vi "y1y2 (子VI)备份.vi"(0 "Image Pixels (U8)输入":u8[][](array[numeric])) -> (7 "left":cluster{i32, i32}[](graph), 8 "right":cluster{i32, i32}[](graph))   [LabVIEW 2014]
panel:
  out "Image Pixels (U8)输入 2":u8[][](array[numeric])
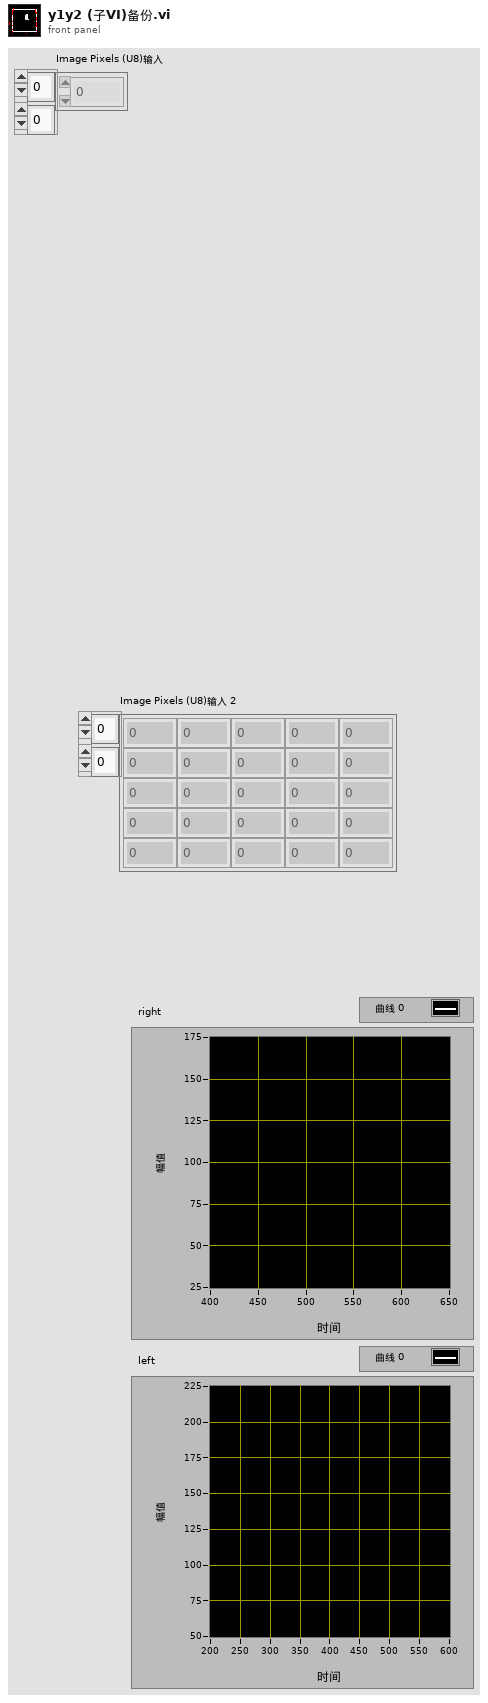
[diagram p1: front panel]
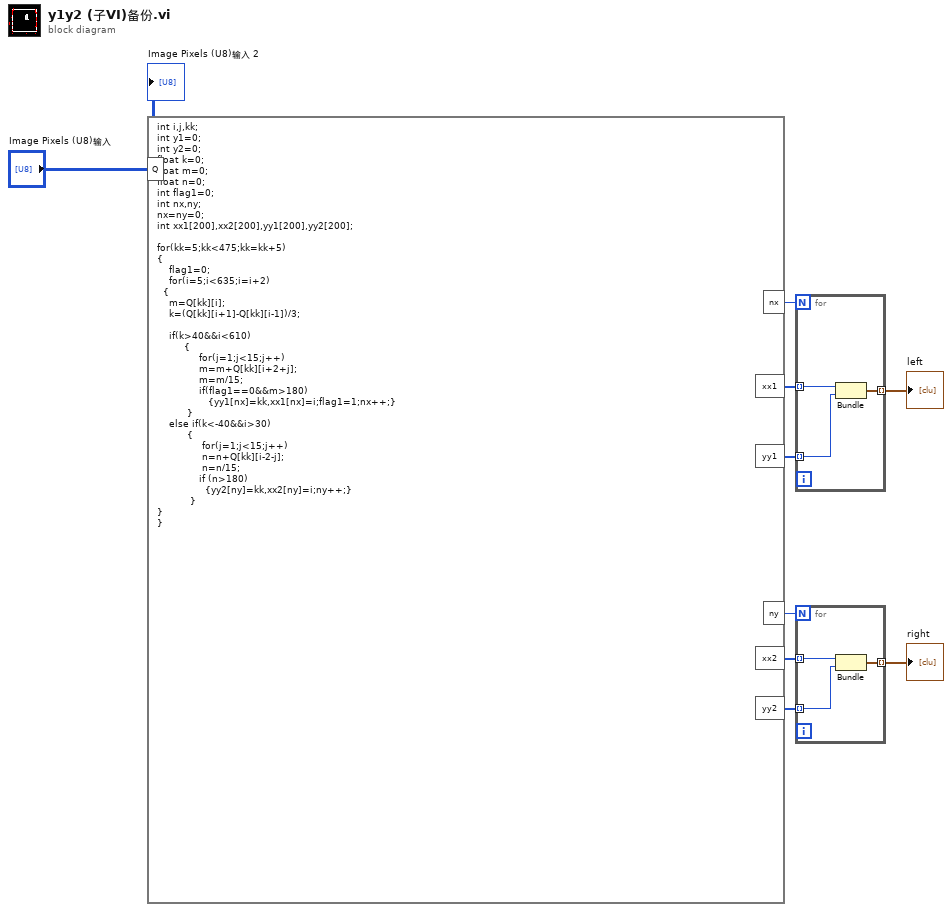
[diagram p0: block diagram]
diagram:
  n1 = formula code="int i,j,kk;\nint y1=0;\nint y2=0;\nfloat k=0;\nfloat m=0;\nfloat n=0;\nint flag1=0;\nint nx,ny;\nnx=ny=0;\nint xx1[200],xx2[200],yy1[200],yy2[200];\n\nfor(kk=5;kk<475;kk=kk+5)\n{\n    flag1=0;\n    for(i=5;i<635;i=i+2)\n  {\n    m=Q[kk][i];\n    k=(Q[kk][i+1]-Q[kk][i-1])/3;\n\n    if(k>40&&i<610)\n         {   \n              for(j=1;j<15;j++)\n              m=m+Q[kk][i+2+j];\n              m=m/15;\n              if(flag1==0&&m>180)\n                 {yy1[nx]=kk,xx1[nx]=i;flag1=1;nx++;}\n          }\n    else if(k<-40&&i>30)\n          {                   \n               for(j=1;j<15;j++)\n               n=n+Q[kk][i-2-j];\n               n=n/15;\n              if (n>180)\n                {yy2[ny]=kk,xx2[ny]=i;ny++;}\n           }\n}\n}"("Q"="Image Pixels (U8)输入") -> ("xx1"=w2:i32[], "yy1"=w1:i32[], "nx"=w3:i32, "xx2"=w4:i32[], "yy2"=w5:i32[], "ny"=w8:i32)
  n2 = for {
    N: w3 -> [_]
    tunnel: w2 -> [w12] mode=indexing
    tunnel: w1 -> [w11] mode=indexing
    tunnel: [w10] -> w6 mode=indexing
    n3 = Bundle(w12, w11) -> (w10:cluster{i32, i32})  [unwired: 1 in]
  }
  "left" <- w6
  n4 = for {
    N: w8 -> [_]
    tunnel: w4 -> [w15] mode=indexing
    tunnel: w5 -> [w14] mode=indexing
    tunnel: [w13] -> w7 mode=indexing
    n5 = Bundle(w15, w14) -> (w13:cluster{i32, i32})  [unwired: 1 in]
  }
  "right" <- w7
  "Image Pixels (U8)输入 2" <- "Image Pixels (U8)输入"
